vi "Set ObjectType.vi"(8 "error in":errorcluster, 10 "ObjectType":refnum<class "Value.lvclass">, 11 "Object Type in":refnum<class "VAR.lvclass">) -> (0 "error out":errorcluster, 3 "Object Type out":refnum<class "VAR.lvclass">)   [LabVIEW 2024, in "Electronic Datasheet.lvlib" / "VAR.lvclass"]
uses:
  VAR.lvclass
  Value/Value.lvclass
  Object Type/Object Type Base.lvclass
  VAR.lvclass/VAR.ctl
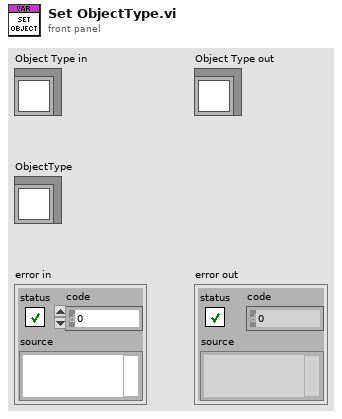
[diagram p1: front panel]
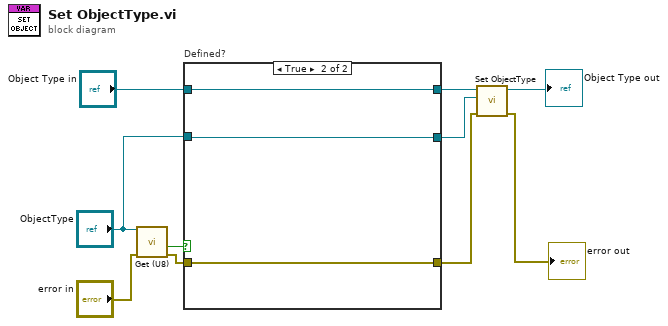
[diagram p0: block diagram]
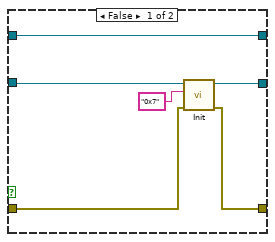
[diagram p2: hidden frame]
diagram:
  n1 = call "Get (U8).vi"("error in"="error in", "Value in"="ObjectType") -> ("error out"=w9:errorcluster, "Defined?"=w10:bool)  [unwired: 6 in, 2 out]
  n2 = case "Defined?" shown="True" w10 {
    tunnel: [w16 w19] -> w2
    tunnel: "Object Type in" -> [w16 w19]
    tunnel: w9 -> [w12 w17]
    tunnel: [w11 w17] -> w3
    tunnel: "ObjectType" -> [w13 w18]
    tunnel: [w15 w18] -> w5
    frame False {
      n3 = call "Init.vi"("error in"=w12, "Value"="0x7", "Value in"=w13) -> ("error out"=w11:errorcluster, "Value out"=w15:refnum<class "Value.lvclass">)  [unwired: 7 in]
    }
    frame True {
    }
  }
  n4 = call-parent "Set ObjectType.vi"("error in"=w3, "ObjectType"=w5, "Object Type in"=w2) -> ("error out"=→"error out":errorcluster, "Object Type out"=→"Object Type out":refnum<class "VAR.lvclass">)  [unwired: 7 in]
